vi "Release.vi"(8 "error in (no error)":errorcluster, 11 "Step in":refnum<class "Step.lvclass">) -> (0 "error out":errorcluster)   [LabVIEW 2020, in "TSnax.lvlib" / "Step.lvclass"]
uses:
  Step.lvclass
  Step.lvclass/Step.ctl
  PropertyObject/PropertyObject.lvclass
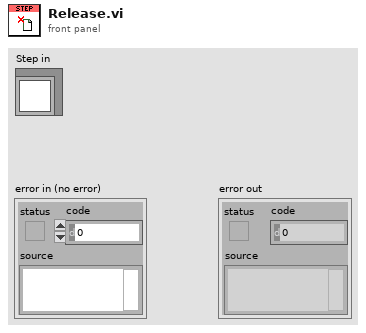
[diagram p1: front panel]
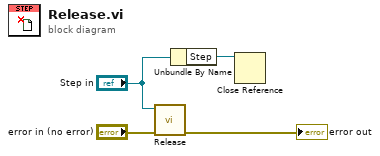
[diagram p0: block diagram]
diagram:
  n1 = call-parent "Release.vi"("error in (no error)"="error in (no error)", "PropertyObject in"="Step in") -> ("error out"=→"error out":errorcluster)  [unwired: 9 in]
  n2 = Unbundle By Name("Step in") -> ("Step"=w1:refnum<k7>)
  n3 = Close Reference(reference=w1) -> ()  [unwired: 1 in, 1 out]
